vi "Conversao_valores_UCM.0200_ENTRADA.vi"(8 "Instrumentos":T3, 11 "UCM.004.EEL.0200_ENTRADA(Controle)":T2) -> (3 "UCM.004.EEL.0200_ENTRADA(Indicador)":T2)   [LabVIEW 2019]
uses:
  padrao_array_cluster_calibracao.ctl
  padrao_UCM.004.EEL.0200_ENTRADA.ctl
panel:
  out "ANALOGICO_entrada":T1
  in  "ANALOGICO_saida":T1
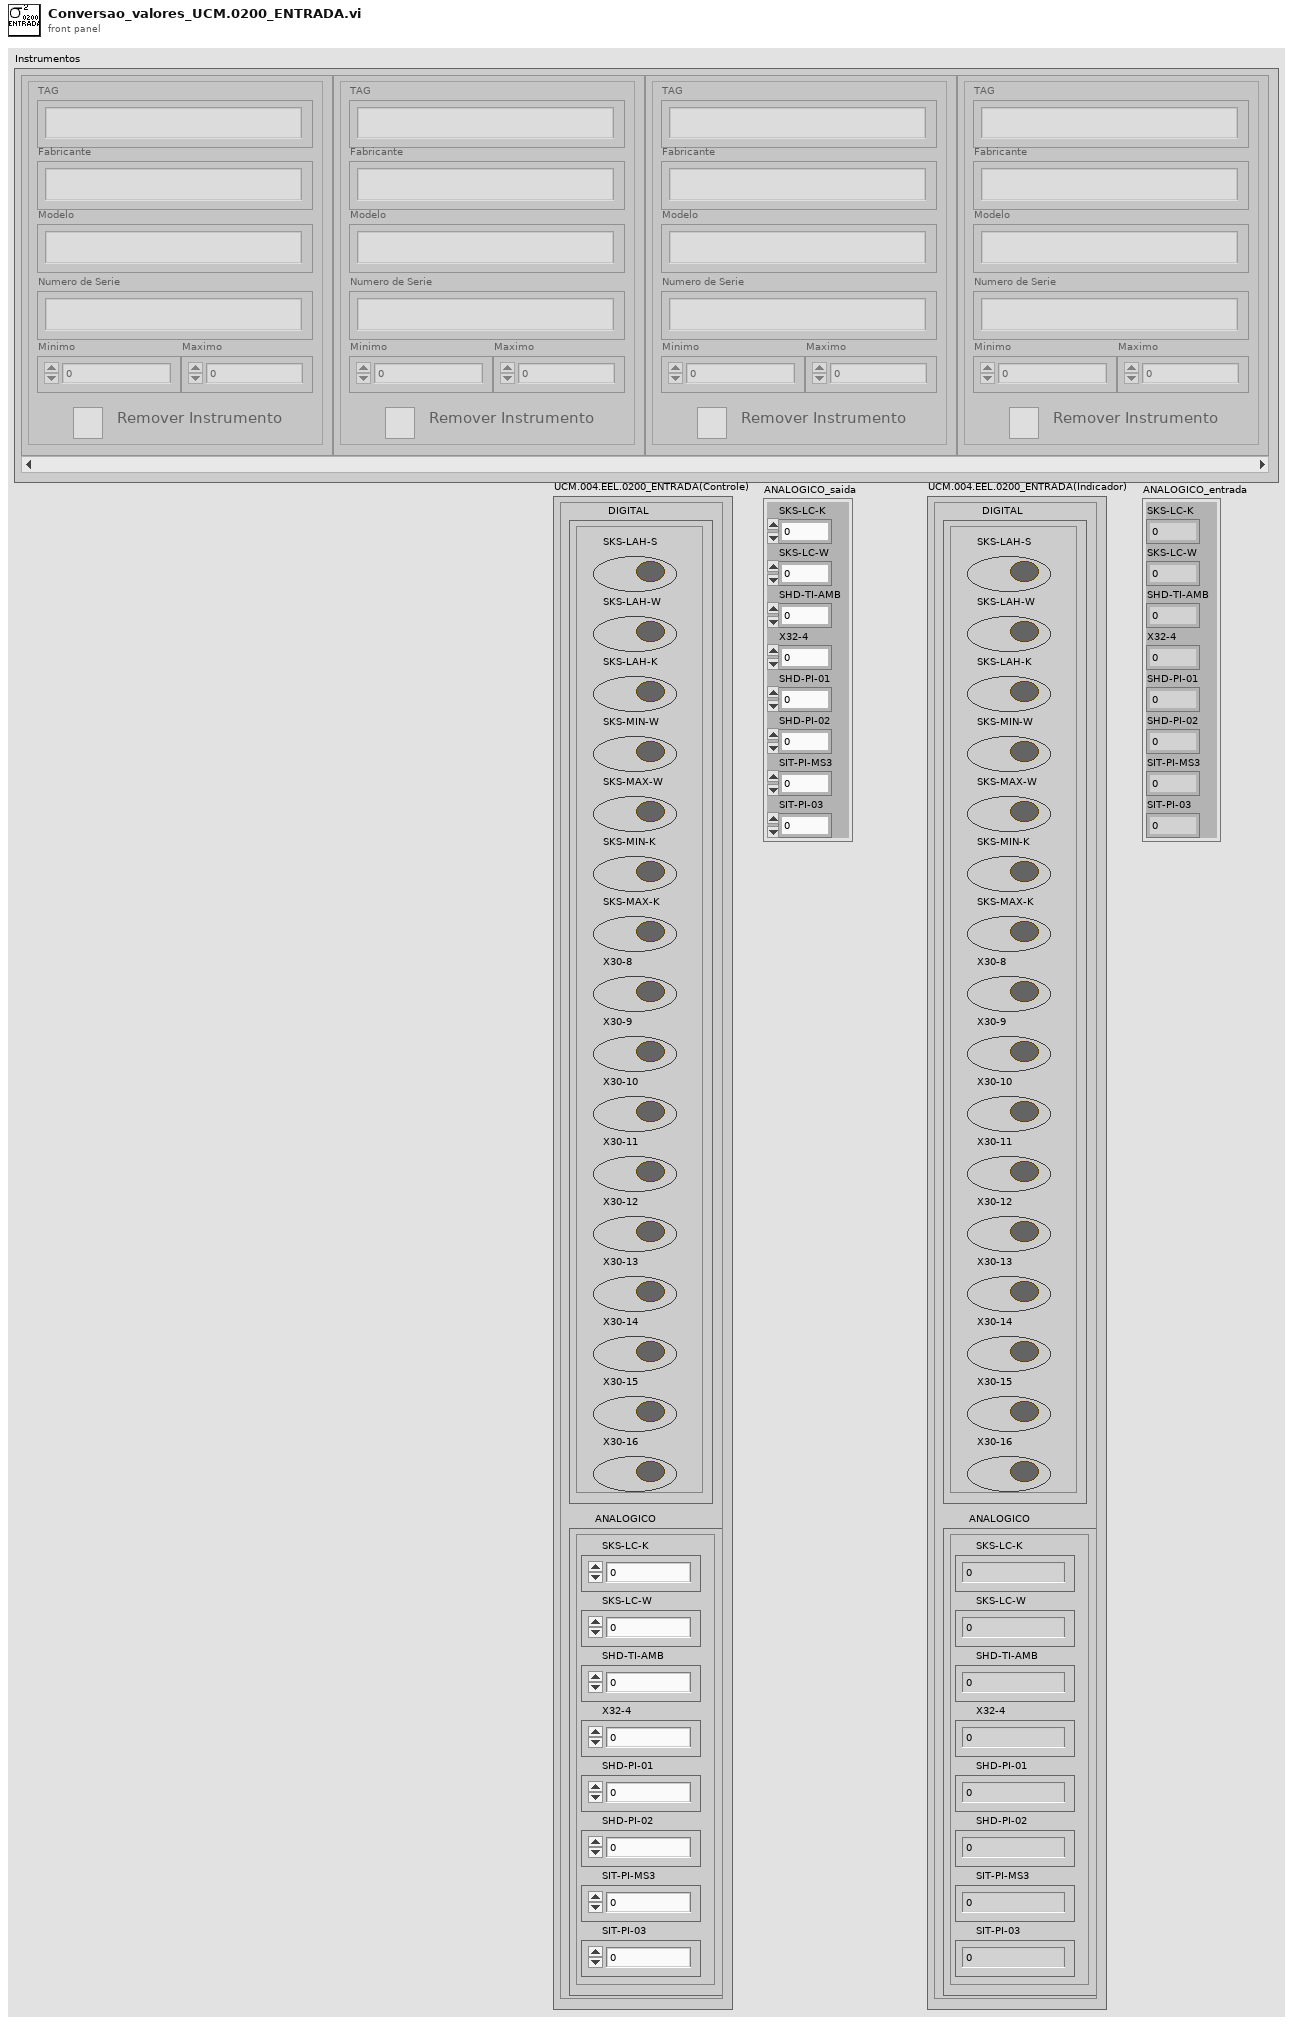
[diagram p1: front panel]
types:
  T1 = cluster{"SKS-LC-K":i16, "SKS-LC-W":i16, "SHD-TI-AMB":i16, "X32-4":i16, "SHD-PI-01":i16, "SHD-PI-02":i16, "SIT-PI-MS3":i16, "SIT-PI-03":i16}
  T2 = typedef "padrao_UCM.004.EEL.0200_ENTRADA.ctl" = cluster{"DIGITAL":cluster{"SKS-LAH-S":bool, "SKS-LAH-W":bool, "SKS-LAH-K":bool, "SKS-MIN-W":bool, "SKS-MAX-W":bool, "SKS-MIN-K":bool, "SKS-MAX-K":bool, "X30-8":bool, "X30-9":bool, "X30-10":bool, "X30-11":bool, "X30-12":bool, "X30-13":bool, "X30-14":bool, "X30-15":bool, "X30-16":bool}, "ANALOGICO":cluster{"SKS-LC-K":i16, "SKS-LC-W":i16, "SHD-TI-AMB":i16, "X32-4":i16, "SHD-PI-01":i16, "SHD-PI-02":i16, "SIT-PI-MS3":i16, "SIT-PI-03":i16}}
  T3 = typedef "padrao_array_cluster_calibracao.ctl" = cluster{"TAG":string, "Minimo":dbl, "Fabricante":string, "Maximo":dbl, "remover_dipositvo":bool, "Modelo":string, "Numero de Serie":string}[]
  T4 = cluster{"TAG":string, "Minimo":dbl, "Fabricante":string, "Maximo":dbl, "remover_dipositvo":bool, "Modelo":string, "Numero de Serie":string}
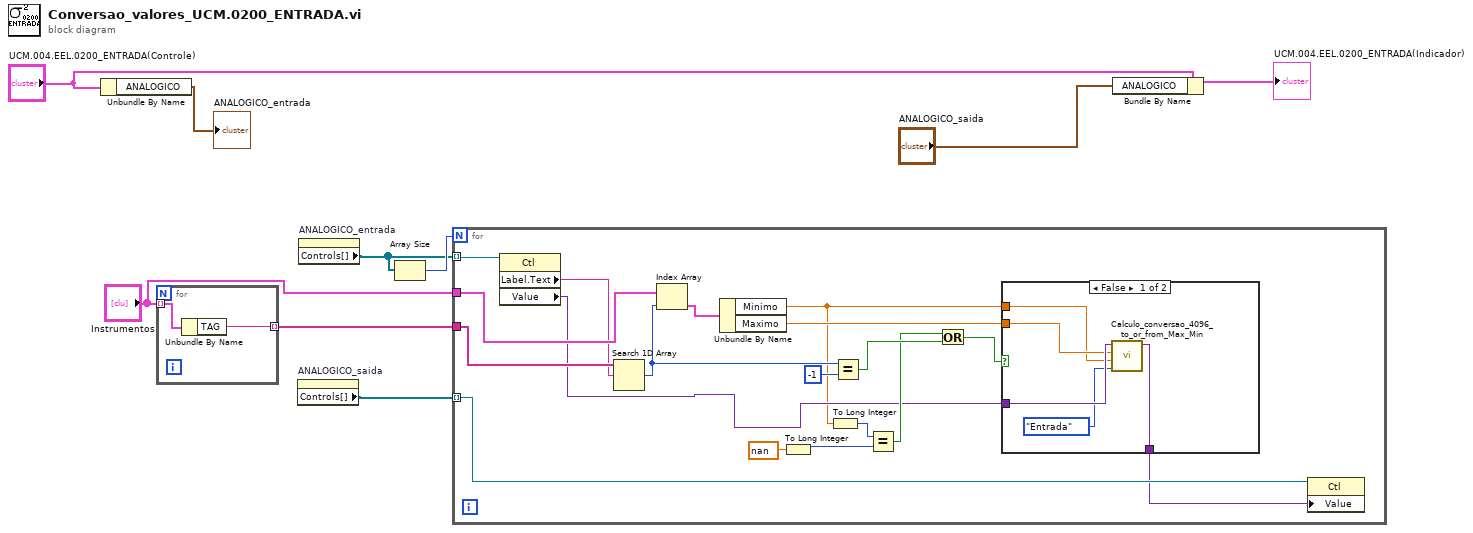
[diagram p0: block diagram]
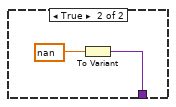
[diagram p2: hidden frame]
diagram:
  n1 = Unbundle By Name("UCM.004.EEL.0200_ENTRADA(Controle)") -> ("ANALOGICO"=→"ANALOGICO_entrada":T1)
  n2 = for {
    tunnel: "Instrumentos" -> [w11] mode=indexing
    tunnel: [w10] -> w9 mode=indexing
    n3 = Unbundle By Name(w11) -> ("TAG"=w10:string)
  }
  n4 = property on="ANALOGICO_saida" class="Clust (strict)"() -> ("Controls[]"=w1:refnum<vi>[])  [unwired: 2 in, 2 out]
  n5 = property on="ANALOGICO_entrada" class="Clust (strict)"() -> ("Controls[]"=w2:refnum<vi>[])  [unwired: 2 in, 2 out]
  n6 = Array Size(array=w2) -> (size(s)=w7:i32)
  n7 = for {
    N: w7 -> [_]
    tunnel: w2 -> [w29] mode=indexing
    tunnel: w1 -> [w25] mode=indexing
    tunnel: w9 -> [w28]
    tunnel: "Instrumentos" -> [w27]
    n8 = property class="Ctl"(reference=w29) -> ("Label.Text"=w24:string, "Value"=w16:variant)  [unwired: 1 in, 2 out]
    n9 = Search 1D Array(1D array=w28, element=w24) -> (index of element=w23:i32)  [unwired: 1 in]
    n10 = Index Array(array=w27, index=w23) -> (element=w26:T4)
    n11 = Unbundle By Name(w26) -> ("Minimo"=w12:dbl, "Maximo"=w13:dbl)
    n12 = To Long Integer(number=nan) -> (32bit integer=w18:i32)
    n13 = To Long Integer(number=w12) -> (32bit integer=w19:i32)
    n14 = Equal?(x=w23, y=-1) -> (x = y?=w21:bool)
    n15 = Equal?(x=w19, y=w18) -> (x = y?=w17:bool)
    n16 = Or(x=w17, y=w21) -> (x .or. y?=w15:bool)
    n17 = case shown="False" w15 {
      tunnel: w16 -> [w34 _]
      tunnel: [w33 w35] -> w14
      tunnel: w13 -> [w31 _]
      tunnel: w12 -> [w30 _]
      frame False {
        n18 = call "Calculo_conversao_4096_to_or_from_Max_Min.vi"("Tipo"=enum16{"Saida", "Entrada"}."Entrada", "Min"=w30, "Max"=w31, "Value"=w34) -> ("Value 2"=w33:variant)  [unwired: 7 in]
      }
      frame True {
        n19 = To Variant(anything=nan) -> (Variant=w35:variant)
      }
    }
    n20 = property class="Ctl"(reference=w25, "Value"=w14) -> ()  [unwired: 1 in, 2 out]
  }
  n21 = Bundle By Name(cluster="UCM.004.EEL.0200_ENTRADA(Controle)", "ANALOGICO"="ANALOGICO_saida") -> (→"UCM.004.EEL.0200_ENTRADA(Indicador)":T2)
